vi "load_udc_config_file.vi"(2 "UDC Table":string[][](array[string]), 3 "Config File":path) -> (0 "Cancelled":bool, 1 "Array":dbl[](array[numeric]))   [LabVIEW 2011]
panel:
  out "Error Out":errorcluster caption="error out"
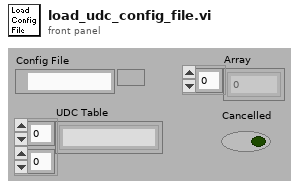
[diagram p1: front panel]
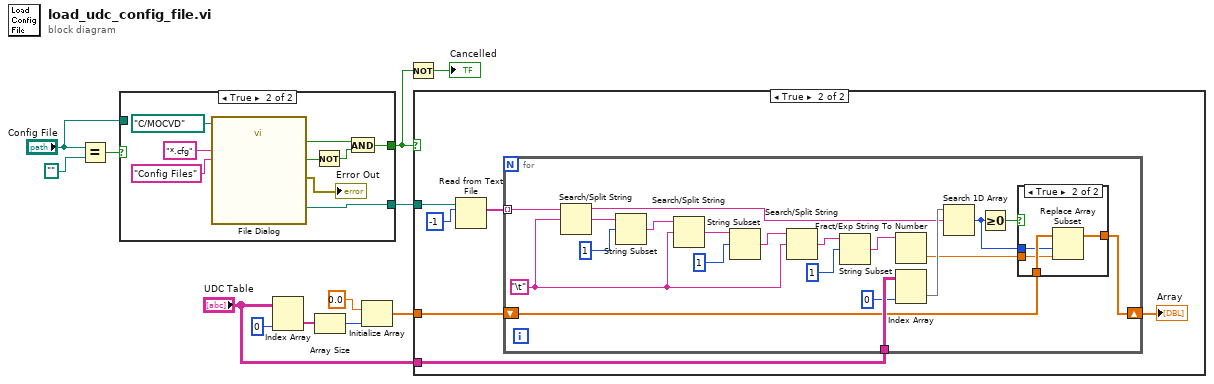
[diagram p0: block diagram]
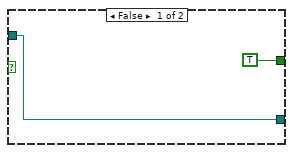
[diagram p4: hidden frame]
diagram:
  n1 = Equal?(x="Config File", y=path "") -> (x = y?=w11:bool)
  n2 = case shown="True" w11 {
    tunnel: [TRUE w15] -> w2
    tunnel: [w14 w19] -> w10
    tunnel: "Config File" -> [w14 _]
    frame False {
    }
    frame True {
      n3 = call "File Dialog"("start path"=path "C:/MOCVD", "pattern (all files)"="*.cfg", "pattern label"="Config Files") -> ("selected path"=w19:path, "exists"=w17:bool, "cancelled"=w20:bool, "error out"=→"Error Out":errorcluster)  [unwired: 4 in, 5 out]
      n4 = Not(x=w20) -> (.not. x?=w16:bool)
      n5 = And(x=w17, y=w16) -> (x .and. y?=w15:bool)
    }
  }
  n6 = Index Array(array="UDC Table", index (col)=0 ("disabled index (col)")) -> (element=w7:string[])  [unwired: 1 in]
  n7 = Array Size(array=w7) -> (size(s)=w6:i32)
  n8 = Initialize Array(0.0 ("element"), w6) -> (w3:dbl[])
  n9 = Not(x=w2) -> (.not. x?=→"Cancelled":bool)
  n10 = case shown="True" w2 {
    tunnel: w10 -> [_ w29]
    tunnel: "UDC Table" -> [_ w26]
    tunnel: w3 -> [_ w25]
    frame False {
    }
    frame True {
      n11 = Read from Text File(file (use dialog)=w29, count=-1) -> (text=w27:string[])  [unwired: 1 in, 4 out]
      n12 = for {
        tunnel: w27 -> [w49] mode=indexing
        tunnel: w26 -> [w41]
        shift-right: [w34] -> w24
        shift-left: w25 -> [w33]
        w43 = "\t"
        n13 = Search/Split String(string=w49, search string/char (-)=w43) -> (substring before match=w30:string, match + rest of string=w32:string)  [unwired: 2 out]
        n14 = String Subset(string=w32, offset (0)=1) -> (substring=w31:string)  [unwired: 1 out]
        n15 = Search/Split String(string=w31, search string/char (-)=w43) -> (match + rest of string=w47:string)  [unwired: 3 out]
        n16 = String Subset(string=w47, offset (0)=1) -> (substring=w48:string)  [unwired: 1 out]
        n17 = Search/Split String(string=w48, search string/char (-)=w43) -> (match + rest of string=w46:string)  [unwired: 3 out]
        n18 = String Subset(string=w46, offset (0)=1) -> (substring=w36:string)  [unwired: 1 out]
        n19 = Fract/Exp String To Number(string=w36) -> (number=w35:dbl)  [unwired: 4 out]
        n20 = Index Array(array=w41, index (col)=0 ("disabled index (col)")) -> (element=w39:string[])  [unwired: 1 in]
        n21 = Search 1D Array(1D array=w39, element=w30) -> (index of element=w37:i32)  [unwired: 1 out]
        n22 = Greater Or Equal To 0?(x=w37) -> (x >= 0?=w38:bool)
        n23 = case shown="True" w38 {
          tunnel: w33 -> [w50 w54]
          tunnel: w37 -> [_ w53]
          tunnel: w35 -> [_ w52]
          tunnel: [w50 w51] -> w34
          frame False {
          }
          frame True {
            n24 = Replace Array Subset(array=w54, new element=w52, index=w53) -> (w51:dbl[])
          }
        }
      }
      "Array" <- w24
    }
  }
